vi "SetJogType.vi"(8 "Error In":errorcluster, 10 "JogMode":i16(ring)=1 items=["ContinuousHeld"=1, "SingleStep"=2, "ContinuousUnheld"=3], 11 "Thorlabs in":refnum<class "Thorlabs.lvclass">) -> (0 "Error Out":errorcluster, 3 "Thorlabs out":refnum<class "Thorlabs.lvclass">)   [LabVIEW 2018, in "Thorlabs.lvlib" / "Thorlabs.lvclass"]
doc: "This VI sets the current jog mode on the Axis Controller.\n\nCreator: Slade Jeppesen\nCreated: 10/02/20"
uses:
  Thorlabs.lvclass
  Thorlabs.lvclass/Thorlabs.ctl
  C:/AME Test Engineering/LabVIEW/PPLs/Axis/DLLs/ThorLabs.MotionControl.KCube.DCServoCLI.dll
  PPLs/Axis/DLLs/ThorLabs.MotionControl.KCube.DCServoCLI.dll
  C:/AME Test Engineering/LabVIEW/PPLs/Axis/DLLs/Thorlabs.MotionControl.GenericMotorCLI.dll
  PPLs/Axis/DLLs/Thorlabs.MotionControl.GenericMotorCLI.dll
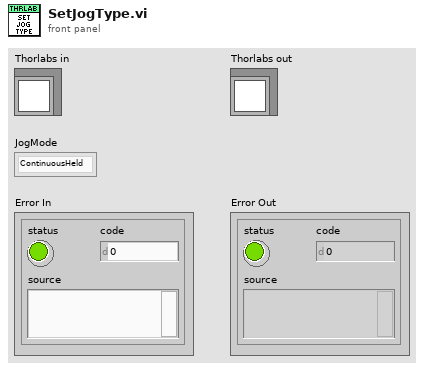
[diagram p1: front panel]
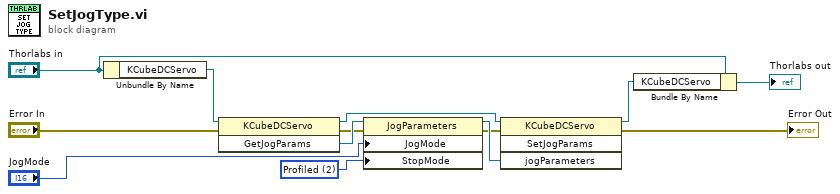
[diagram p0: block diagram]
diagram:
  w1 = i16 2 items=["Immediate"=1, "Profiled"=2] ("StopMode")
  n1 = Unbundle By Name("Thorlabs in") -> ("KCubeDCServo"=w13:refnum<k24>)
  n2 = invoke class="KCubeDCServo" method="GetJogParams"(reference=w13, error in="Error In") -> (reference out=w10:refnum<k24>, error out=w11:errorcluster, "GetJogParams"=w12:refnum<k24>)  [unwired: 1 in]
  n3 = property class="JogParameters"(reference=w12, error in=w11, "JogMode"="JogMode", "StopMode"=w1) -> (reference out=w9:refnum<k24>, error out=w8:errorcluster)
  n4 = invoke class="KCubeDCServo" method="SetJogParams"(reference=w10, error in=w8, "jogParameters"=w9) -> (reference out=w5:refnum<k24>, error out=→"Error Out":errorcluster)  [unwired: 1 in, 2 out]
  n5 = Bundle By Name(cluster="Thorlabs in", "KCubeDCServo"=w5) -> (→"Thorlabs out":refnum<class "Thorlabs.lvclass">)
